vi "Populate.vi"(0 "Path":path, 11 "Error in":errorcluster) -> (4 "Tree":string(tree), 15 "Error out":errorcluster)   [LabVIEW 2020]
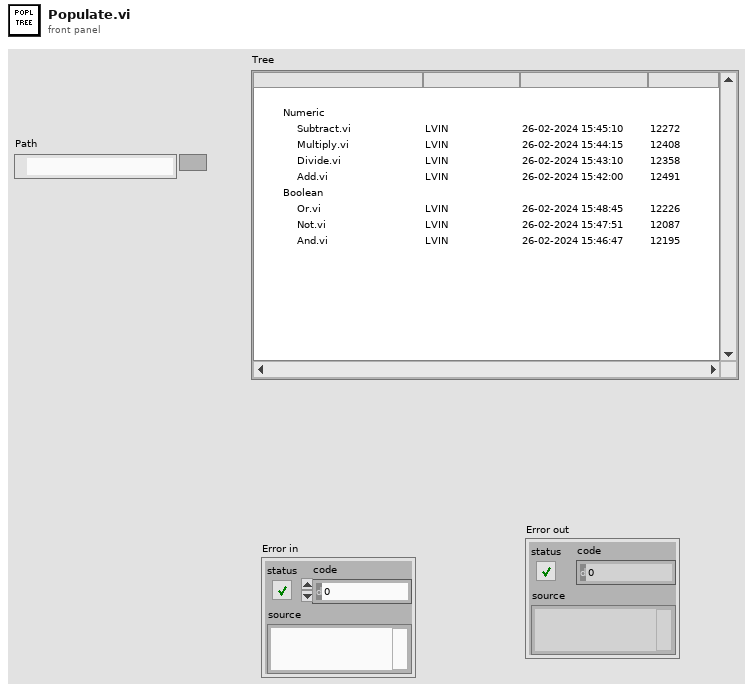
[diagram p1: front panel]
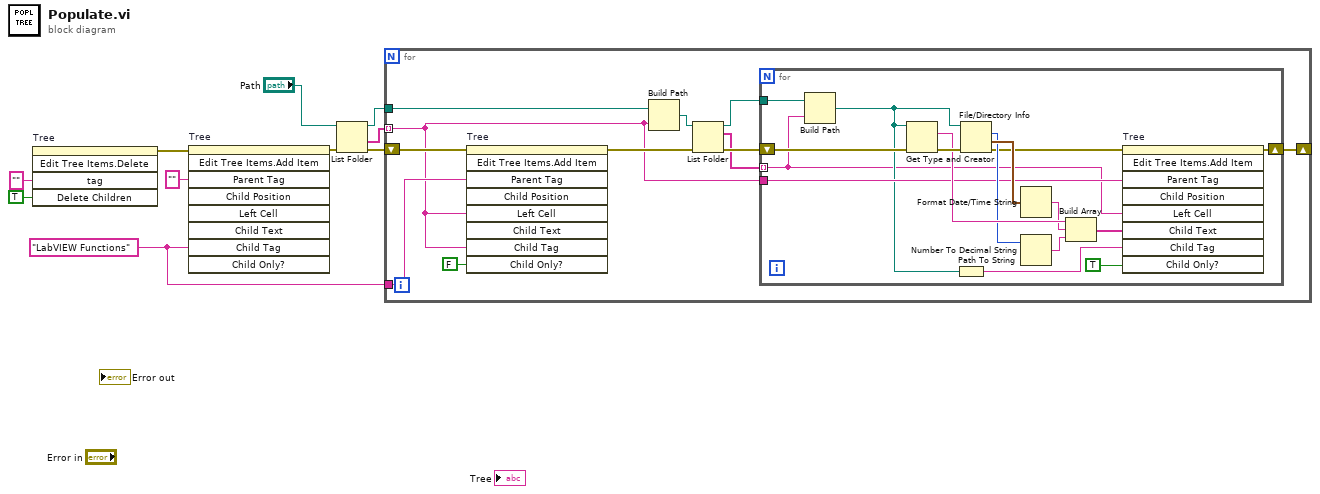
[diagram p0: block diagram]
diagram:
  w2 = "LabVIEW Functions" ("Child Tag")
  n1 = invoke on="Tree" class="Tree (strict)" method="Edit Tree Items.Delete"("tag"="" ("Tag"), "Delete Children"=TRUE ("Delete Children?")) -> (error out=w8:errorcluster)  [unwired: 3 in, 4 out]
  n2 = invoke on="Tree" class="Tree (strict)" method="Edit Tree Items.Add Item"(error in=w8, "Parent Tag"="", "Child Tag"=w2) -> (error out=w5:errorcluster)  [unwired: 6 in, 8 out]
  n3 = List Folder(path="Path", error in=w5) -> (path out=w3:path, folder names=w4:string[], error out=w6:errorcluster)  [unwired: 2 in, 1 out]
  n4 = for {
    tunnel: w3 -> [w17]
    shift-right: [w21] -> _
    shift-left: w6 -> [w20]
    tunnel: w4 -> [w11] mode=indexing
    tunnel: w2 -> [w19]
    n5 = invoke on="Tree" class="Tree (strict)" method="Edit Tree Items.Add Item"(error in=w20, "Parent Tag"=w19, "Left Cell"=w11, "Child Tag"=w11, "Child Only?"=FALSE) -> (error out=w16:errorcluster)  [unwired: 4 in, 8 out]
    n6 = Build Path(base path=w17, name or relative path=w11) -> (appended path=w14:path)
    n7 = List Folder(path=w14, error in=w16) -> (path out=w13:path, filenames=w12:string[], error out=w15:errorcluster)  [unwired: 2 in, 1 out]
    n8 = for {
      tunnel: w13 -> [w23]
      tunnel: w11 -> [w28]
      shift-right: [w29] -> w21
      shift-left: w15 -> [w31]
      tunnel: w12 -> [w22] mode=indexing
      n9 = Build Path(base path=w23, name or relative path=w22) -> (appended path=w24:path)
      n10 = Get Type and Creator(4:w31, 7:w24) -> (0:w37:errorcluster, 2:w36:string)  [unwired: 2 out]
      n11 = Path To String(path=w24) -> (string=w26:string)
      n12 = File/Directory Info(path=w24, error in=w37) -> (size=w33:i64, last mod=w35:timestamp, error out=w30:errorcluster)  [unwired: 4 out]
      n13 = Format Date/Time String(seconds (now)=w35) -> (date/time string=w34:string)  [unwired: 2 in]
      n14 = Number To Decimal String(number=w33) -> (decimal integer string=w32:string)  [unwired: 1 in]
      n15 = Build Array(w36, w34, w32) -> (w25:string[])
      n16 = invoke on="Tree" class="Tree (strict)" method="Edit Tree Items.Add Item"(error in=w30, "Parent Tag"=w28, "Left Cell"=w22, "Child Text"=w25, "Child Tag"=w26, "Child Only?"=TRUE) -> (error out=w29:errorcluster)  [unwired: 3 in, 8 out]
    }
  }
